vi "parse_depth_data.vi"(4 "error in":errorcluster, 6 "Distance (meters)":sgl[unit](slide)=46.464645 scale=0.0..100.0, 7 "Data":string) -> (0 "error out":errorcluster, 2 "Normalized data":u8[](array[numeric]), 3 "Raw data":sgl[](array[numeric]))   [LabVIEW 2019, in "Lib_Simx.lvlib"]
doc: "Parse the raw data from the Depth Camera sensor and output the normalized data."
uses:
  Lib_Simx.lvlib
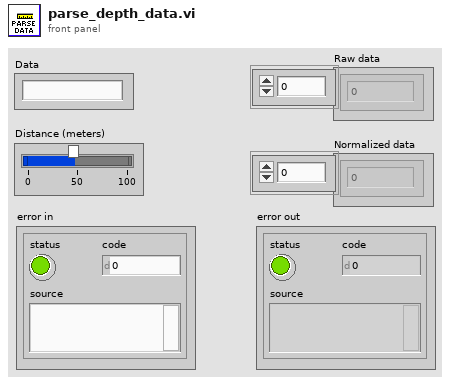
[diagram p1: front panel]
types:
  T1 = enum16{"big-endian, network order", "native, host order", "little-endian"}
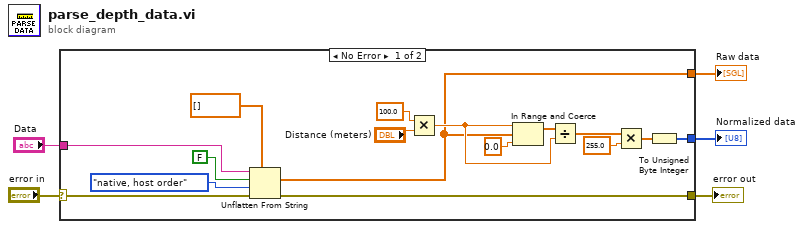
[diagram p0: block diagram]
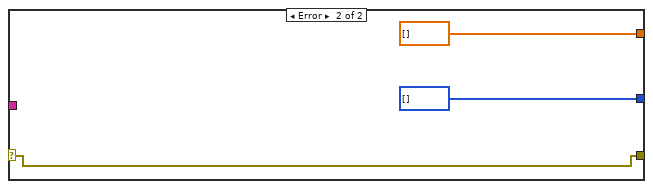
[diagram p2: hidden frame]
diagram:
  n1 = case shown="No Error" "error in" {
    selector: "error in" -> [w6 w24]
    tunnel: [w19 sgl[] []] -> w5
    tunnel: "Data" -> [w18 _]
    tunnel: [w10 u8[] []] -> w3
    tunnel: [w7 w24] -> w1
    frame No Error {
      n2 = Unflatten From String(type=sgl[] [], binary string=w18, data includes array or string size? (T)=FALSE, byte order (0:big-endian, network order)=T1."native, host order", error in (no error)=w6) -> (value=w19:sgl[], error out=w7:errorcluster)  [unwired: 1 out]
      n3 = Multiply(x=sgl 100.0, y="Distance (meters)") -> (x*y=w20:sgl[unit])
      n4 = In Range and Coerce(upper limit=w20, x=w19, lower limit=sgl 0.0) -> (coerced(x)=w11:sgl[unit][])  [unwired: 1 out]
      n5 = Divide(x=w11, y=w20) -> (x/y=w12:sgl[])
      n6 = Multiply(x=w12, y=sgl 255.0) -> (x*y=w14:sgl[])
      n7 = To Unsigned Byte Integer(number=w14) -> (unsigned 8bit integer=w10:u8[])
    }
    frame Error {
    }
  }
  "Raw data" <- w5
  "Normalized data" <- w3
  "error out" <- w1
